vi "ST4 current buffer.vi"(7 "Mode":enum16{"Read", "Write"}(ring)=enum."Write", 10 "index":i32, 11 "in":dbl[](array[numeric])) -> (2 "out":dbl, 3 "out(ALL)":dbl[](array[numeric]))   [LabVIEW 2018]
panel:
  out "data out":sgl
  in  "data in":sgl[](array[numeric])
  in  "Mode":enum16{"Initialize", "Read", "Write"}(ring)=enum."Read"
  in  "staion index":i32
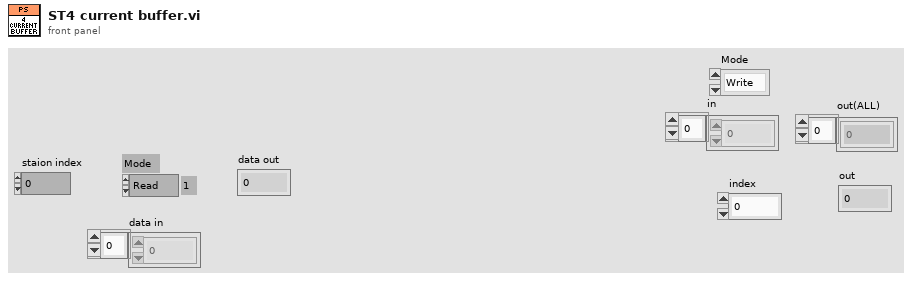
[diagram p1: front panel]
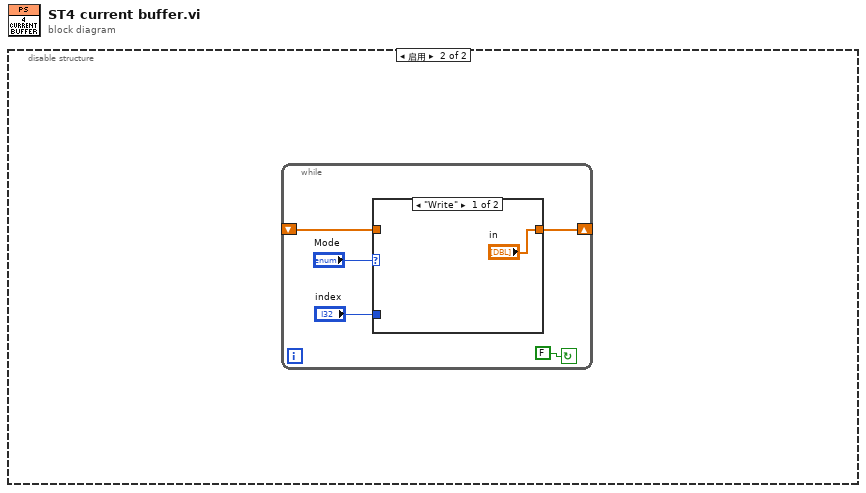
[diagram p0: block diagram]
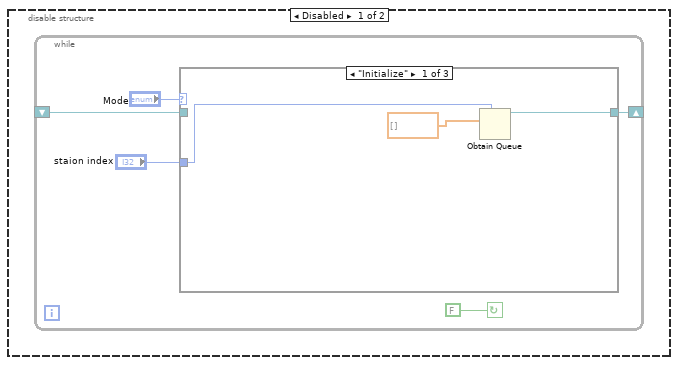
[diagram p2: hidden frame]
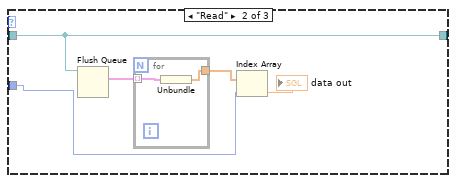
[diagram p3: hidden frame]
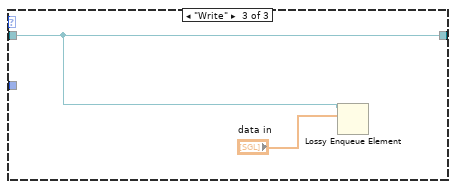
[diagram p4: hidden frame]
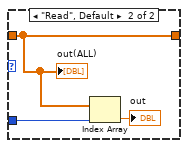
[diagram p5: hidden frame]
diagram:
  n1 = disable-structure shown="启用" {
    frame Disabled {
      n2 = while {
        shift-right: [w3] -> _
        shift-left: _ -> [w2]
        stop <- FALSE continue-if-true
        n3 = case shown="\"Initialize\"" "Mode" {
          tunnel: [w8 w13 w17] -> w3
          tunnel: w2 -> [_ w13 w17]
          tunnel: "staion index" -> [w6 w9 _]
          frame "Initialize" {
            n4 = Obtain Queue(max queue size (-1, unlimited)=w6, element data type=sgl[] []) -> (queue out=w8:refnum<queue>)  [unwired: 3 in, 2 out]
          }
          frame "Read" {
            n5 = Flush Queue(queue=w13) -> (remaining elements=w12:cluster{sgl[]}[])  [unwired: 1 in, 2 out]
            n6 = for {
              tunnel: w12 -> [w15] mode=indexing
              tunnel: [w14] -> w11
              n7 = Unbundle(w15) -> (w14:sgl[])
            }
            n8 = Index Array(array=w11, index=w9) -> (element=→"data out":sgl)
          }
          frame "Write" {
            n9 = Lossy Enqueue Element(queue=w17, element="data in") -> ()  [unwired: 1 in, 4 out]
          }
        }
      }
    }
    frame Enabled {
      n10 = while {
        shift-right: [w20] -> _
        shift-left: _ -> [w22]
        stop <- FALSE continue-if-true
        n11 = case shown="\"Write\"" "Mode" {
          tunnel: w22 -> [_ w26]
          tunnel: ["in" w26] -> w20
          tunnel: "index" -> [_ w25]
          frame "Write" {
          }
          frame "Read", Default {
            n12 = Index Array(array=w26, index=w25) -> (element=→"out":dbl)
            "out(ALL)" <- w26
          }
        }
      }
    }
  }
